vi "Forcade_Picture_Size_Get.vi"(8 "error in (no error)":errorcluster caption="错误输入（无错误）", 11 "Picture_Class 输入":refnum<class "Picture_Class.lvclass"> caption="DNL_LabVIEW Object in") -> (0 "error out":errorcluster caption="错误输出", 2 "Picture Size":T1, 3 "Picture_Class 输出":refnum<class "Picture_Class.lvclass"> caption="DNL_LabVIEW Object out")   [LabVIEW 2013, in "Picture_Class.lvclass"]
uses:
  Picture_Class.lvclass
  <vilib>/Utility/miscctls.llb/LVBoundsTypeDef.ctl
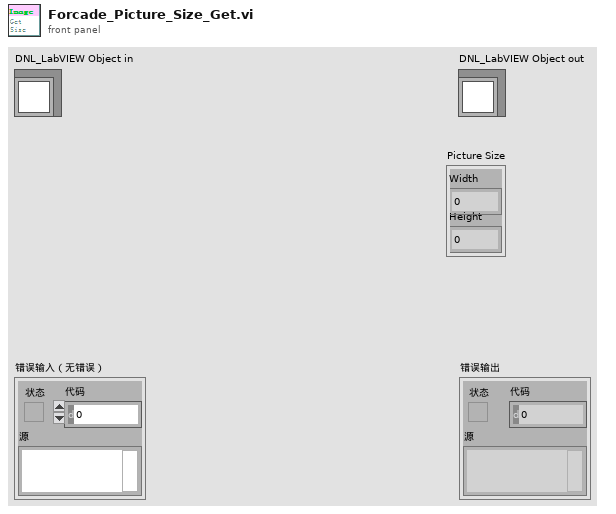
[diagram p1: front panel]
types:
  T1 = typedef "LVBoundsTypeDef.ctl" = cluster{"Width":u32, "Height":u32}
  T2 = typedef "imagedata.ctl" = cluster{"image type":i32, "image depth":i32, "image":u8[], "mask":u8[], "colors":u32[], "Rectangle":cluster{"left":i16, "top":i16, "right":i16, "bottom":i16}}
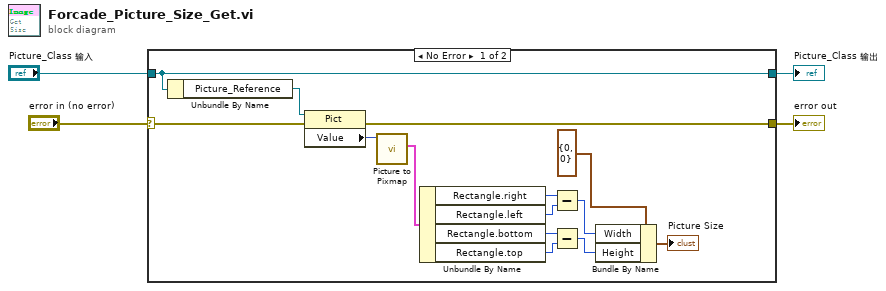
[diagram p0: block diagram]
diagram:
  n1 = case shown="No Error" "error in (no error)" {
    selector: "error in (no error)" -> [w16 w20]
    tunnel: [w15 w20] -> w3
    tunnel: [w18 w19] -> w1
    tunnel: "Picture_Class 输入" -> [w18 w19]
    frame No Error {
      n2 = Unbundle By Name(w18) -> ("Picture_Reference"=w17:refnum<vi>)
      n3 = property class="Pict"(reference=w17, error in=w16) -> (error out=w15:errorcluster, "Value"=w13:picture)  [unwired: 1 out]
      n4 = call <vilib>:"Picture to Pixmap.vi"("picture"=w13) -> ("image data"=w14:T2)  [unwired: 9 in, 1 out]
      n5 = Unbundle By Name(w14) -> ("Rectangle.right"=w12:i16, "Rectangle.left"=w11:i16, "Rectangle.bottom"=w10:i16, "Rectangle.top"=w7:i16)
      n6 = Subtract(x=w12, y=w11) -> (x-y=w8:i16)
      n7 = Subtract(x=w10, y=w7) -> (x-y=w5:i16)
      n8 = Bundle By Name(cluster=T1 {"Width"=0, "Height"=0} ("Draw Area Size 2"), "Width"=w8, "Height"=w5) -> (→"Picture Size":T1)
    }
    frame Error {
    }
  }
  "error out" <- w3
  "Picture_Class 输出" <- w1
